vi "Source-TDMS setup strings.vi"() -> (2 "Functional imaging TDMS channel names array":string[](array[string]), 3 "TDMS group name":string)   [LabVIEW 2020]
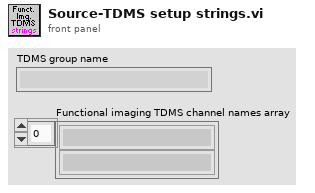
[diagram p1: front panel]
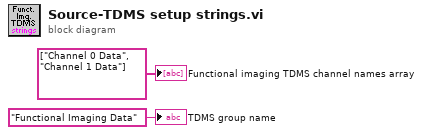
[diagram p0: block diagram]
diagram:
  "Functional imaging TDMS channel names array" <- string[] ["Channel 0 Data", "Channel 1 Data"] ("channel name(s) in (Untitled)")
  "TDMS group name" <- "Functional Imaging Data" ("group name in (Untitled)")
